vi "Read IED Status DVR (DeviceIDs).vi"(8 "error in":errorcluster, 11 "EMS Generic in":refnum<class "EMS Generic.lvclass">) -> (0 "error out":errorcluster, 2 "DeviceID Array":T1[](array[typedef]), 3 "EMS Generic out":refnum<class "EMS Generic.lvclass">)   [LabVIEW 2018, in "EMS Generic Actor.lvlib" / "EMS Generic.lvclass"]
uses:
  EMS Generic.lvclass
  <vilib>/ORNL/CSEISMIC DDS/CSEISMIC DDS Base/Data Types/Controls/DeviceID.ctl
  EMS Generic.lvclass/EMS Generic.ctl
  <vilib>/ORNL/CSEISMIC DDS/CSEISMIC DDS Base/CSEISMIC DDS.lvclass
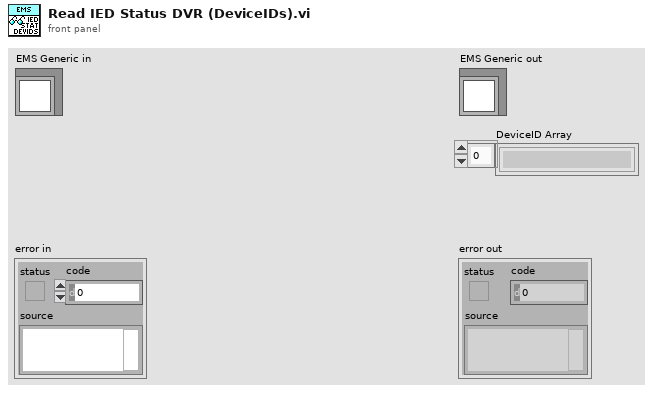
[diagram p1: front panel]
types:
  T1 = typedef "CSEISMIC DDS.lvlib/CSEISMIC DDS.lvclass/DeviceID.ctl" = string
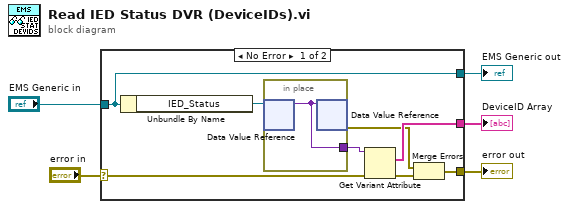
[diagram p0: block diagram]
diagram:
  n1 = case shown="No Error" "error in" {
    selector: "error in" -> [w8 w16]
    tunnel: [w11 w16] -> w2
    tunnel: [w13 w15] -> w3
    tunnel: "EMS Generic in" -> [w13 w15]
    tunnel: [w9 _] -> w1
    frame No Error {
      n2 = Unbundle By Name(w13) -> ("IED_Status"=w12:refnum<data-value>)
      n3 = in-place {
        in-place-border: [w14] -> w10
        n4 = in-place-dvr #1(w12) -> (w14:variant)  [unwired: 1 out]
        n5 = in-place-dvr #1(w14) -> (w6:errorcluster)  [unwired: 1 out]
      }
      n6 = Get Variant Attribute(Variant=w10, error in=w8) -> (names=w9:string[], error out=w7:errorcluster)  [unwired: 2 in, 2 out]
      n7 = Merge Errors(w6, w7) -> (w11:errorcluster)
    }
    frame Error {
    }
  }
  "error out" <- w2
  "EMS Generic out" <- w3
  "DeviceID Array" <- w1
